vi "Create Skipfire Command.vi"(8 "error in (no error)":errorcluster, 11 "Section Ptr":T2 format="%.0x") -> (0 "error out":errorcluster, 3 "Parent Ref out":T2 format="%.0x")   [LabVIEW 2016, in "DCM System Explorer.lvlib"]
uses:
  DCM System Explorer.lvlib
  <vilib>/NI Veristand/Custom Device API/Custom Device Item Ref.ctl
  <vilib>/Powertrain Controls/Device Drivers/DCM/Skip Fire/RT/Skip Fire Setup.ctl
  <vilib>/NI Veristand/Custom Device API/Custom Device Channel Type.ctl
  Shared/DCM Properties.vi
  <vilib>/NI VeriStand/Custom Device API/Custom Device API.lvlib
  DCM Shared.lvlib
  <vilib>/Powertrain Controls/Device Drivers/DCM/Skip Fire/RT/DCM - RT - Skip Fire.lvlib
panel:
  in  "Setup":T1[](array[typedef])=[{"Enable"=FALSE, "Total Cycles"=0, "On Cycles"=0, "TDC Offset [CAD]"=0.0}, {"Enable"=FALSE, "Total Cycles"=0, "On Cycles"=0, "TDC Offset [CAD]"=0.0}, {"Enable"=FALSE, "Total Cycles"=0, "On Cycles"=0, "TDC Offset [CAD]"=0.0}, {"Enable"=FALSE, "Total Cycles"=0, "On Cycles"=0, "TDC Offset [CAD]"=0.0}, {"Enable"=FALSE, "Total Cycles"=0, "On Cycles"=0, "TDC Offset [CAD]"=0.0}, {"Enable"=FALSE, "Total Cycles"=0, "On Cycles"=0, "TDC Offset [CAD]"=0.0}, {"Enable"=FALSE, "Total Cycles"=0, "On Cycles"=0, "TDC Offset [CAD]"=0.0}, {"Enable"=FALSE, "Total Cycles"=0, "On Cycles"=0, "TDC Offset [CAD]"=0.0}]
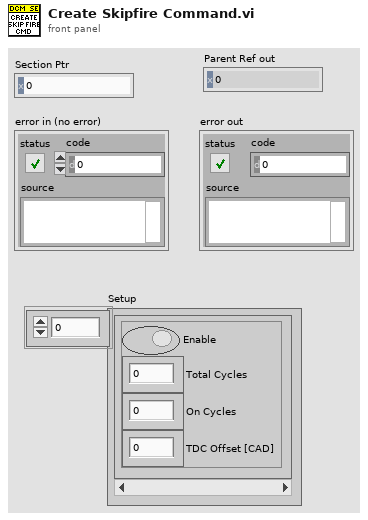
[diagram p1: front panel]
types:
  T1 = typedef "DCM - RT - Skip Fire.lvlib/Skip Fire Setup.ctl" = cluster{"Enable":bool, "Total Cycles":u8, "On Cycles":u8, "TDC Offset [CAD]":sgl}
  T2 = typedef "Custom Device API.lvlib/Custom Device Item Ref.ctl" = u64
  T3 = typedef "Custom Device API.lvlib/Custom Device Channel Type.ctl" = enum16{"Input", "Output"}
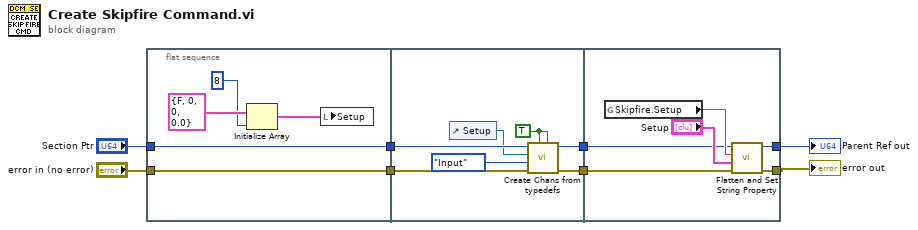
[diagram p0: block diagram]
diagram:
  n1 = flat-sequence {
    tunnel: [w12] -> w7
    tunnel: [w13] -> w8
    tunnel: "error in (no error)" -> [w13]
    tunnel: "Section Ptr" -> [w12]
    tunnel: [w15] -> w6
    tunnel: [w14] -> w5
    tunnel: w8 -> [w18]
    tunnel: w7 -> [w19]
    tunnel: [w26] -> w2
    tunnel: w6 -> [w22]
    tunnel: w5 -> [w21]
    tunnel: [w23] -> w1
    frame #0 {
      n2 = Initialize Array(T1 {"Enable"=FALSE, "Total Cycles"=0, "On Cycles"=0, "TDC Offset [CAD]"=0.0} ("PWM Control 2"), 8 ("dimension size")) -> (w10:T1[])
      n3 = local write "Setup"(w10) -> ()
    }
    frame #1 {
      w17 = TRUE ("Prevent overwrite? (F)")
      n4 = control-ref of="Setup"() -> (w16:refnum<vi>)
      n5 = call "Create Chans from typedefs.vi"("Default from text? (F)"=w17, "Prevent overwrite? (F)"=w17, "error in"=w18, "Type"=Custom_Device_Channel_Type."Input", "Ctl Ref"=w16, "Section Ref in"=w19) -> ("error out"=w14:errorcluster, "Section Ref out"=w15:T2)  [unwired: 3 in, 1 out]
    }
    frame #2 {
      n6 = global read "DCM Properties.vi" "Skipfire.Setup"() -> (w25:string)
      n7 = call "Flatten and Set String Property.vi"("error in (no error)"=w21, "Value"="Setup", "Property Name"=w25, "Section Ref in"=w22) -> ("error out"=w26:errorcluster, "Section Ref out"=w23:T2)  [unwired: 6 in]
    }
  }
  "Parent Ref out" <- w1
  "error out" <- w2
